vi "Door_Access_System.vi"() -> ()   [LabVIEW 2026]
panel:
  out "String":string
  out "s4":i32
  out "s3":i32
  out "s2":i32
  out "s1":i32
  in  "D":bool
  in  "C":bool
  in  "B":bool
  in  "A":bool
  in  "E":bool
  in  "F":bool
  in  "9":bool
  in  "8":bool
  in  "7":bool
  in  "6":bool
  in  "5":bool
  in  "4":bool
  in  "3":bool
  in  "2":bool
  in  "1":bool
  in  "0":bool
  in  "stop 3":bool
  in  "stop 2":bool
  in  "Digits":i32
  out "7-segment":T1
  in  "stop":bool
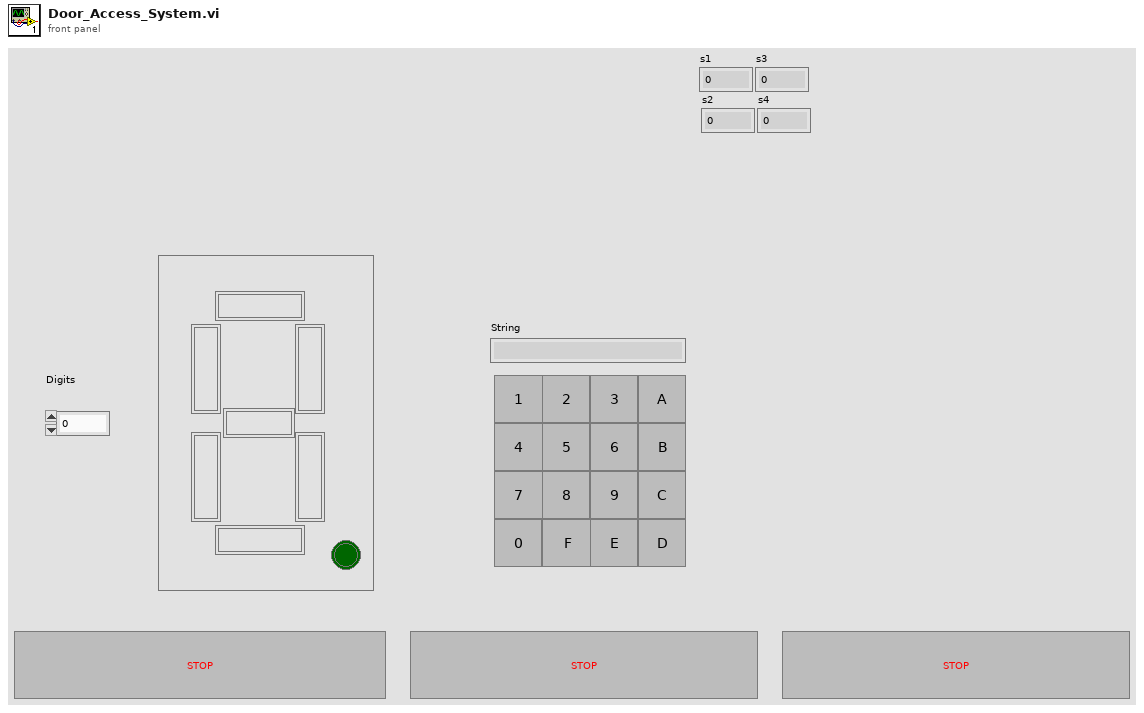
[diagram p1: front panel]
types:
  T1 = cluster{"a":bool, "b":bool, "c":bool, "d":bool, "e":bool, "f":bool, "g":bool, "DP":bool}
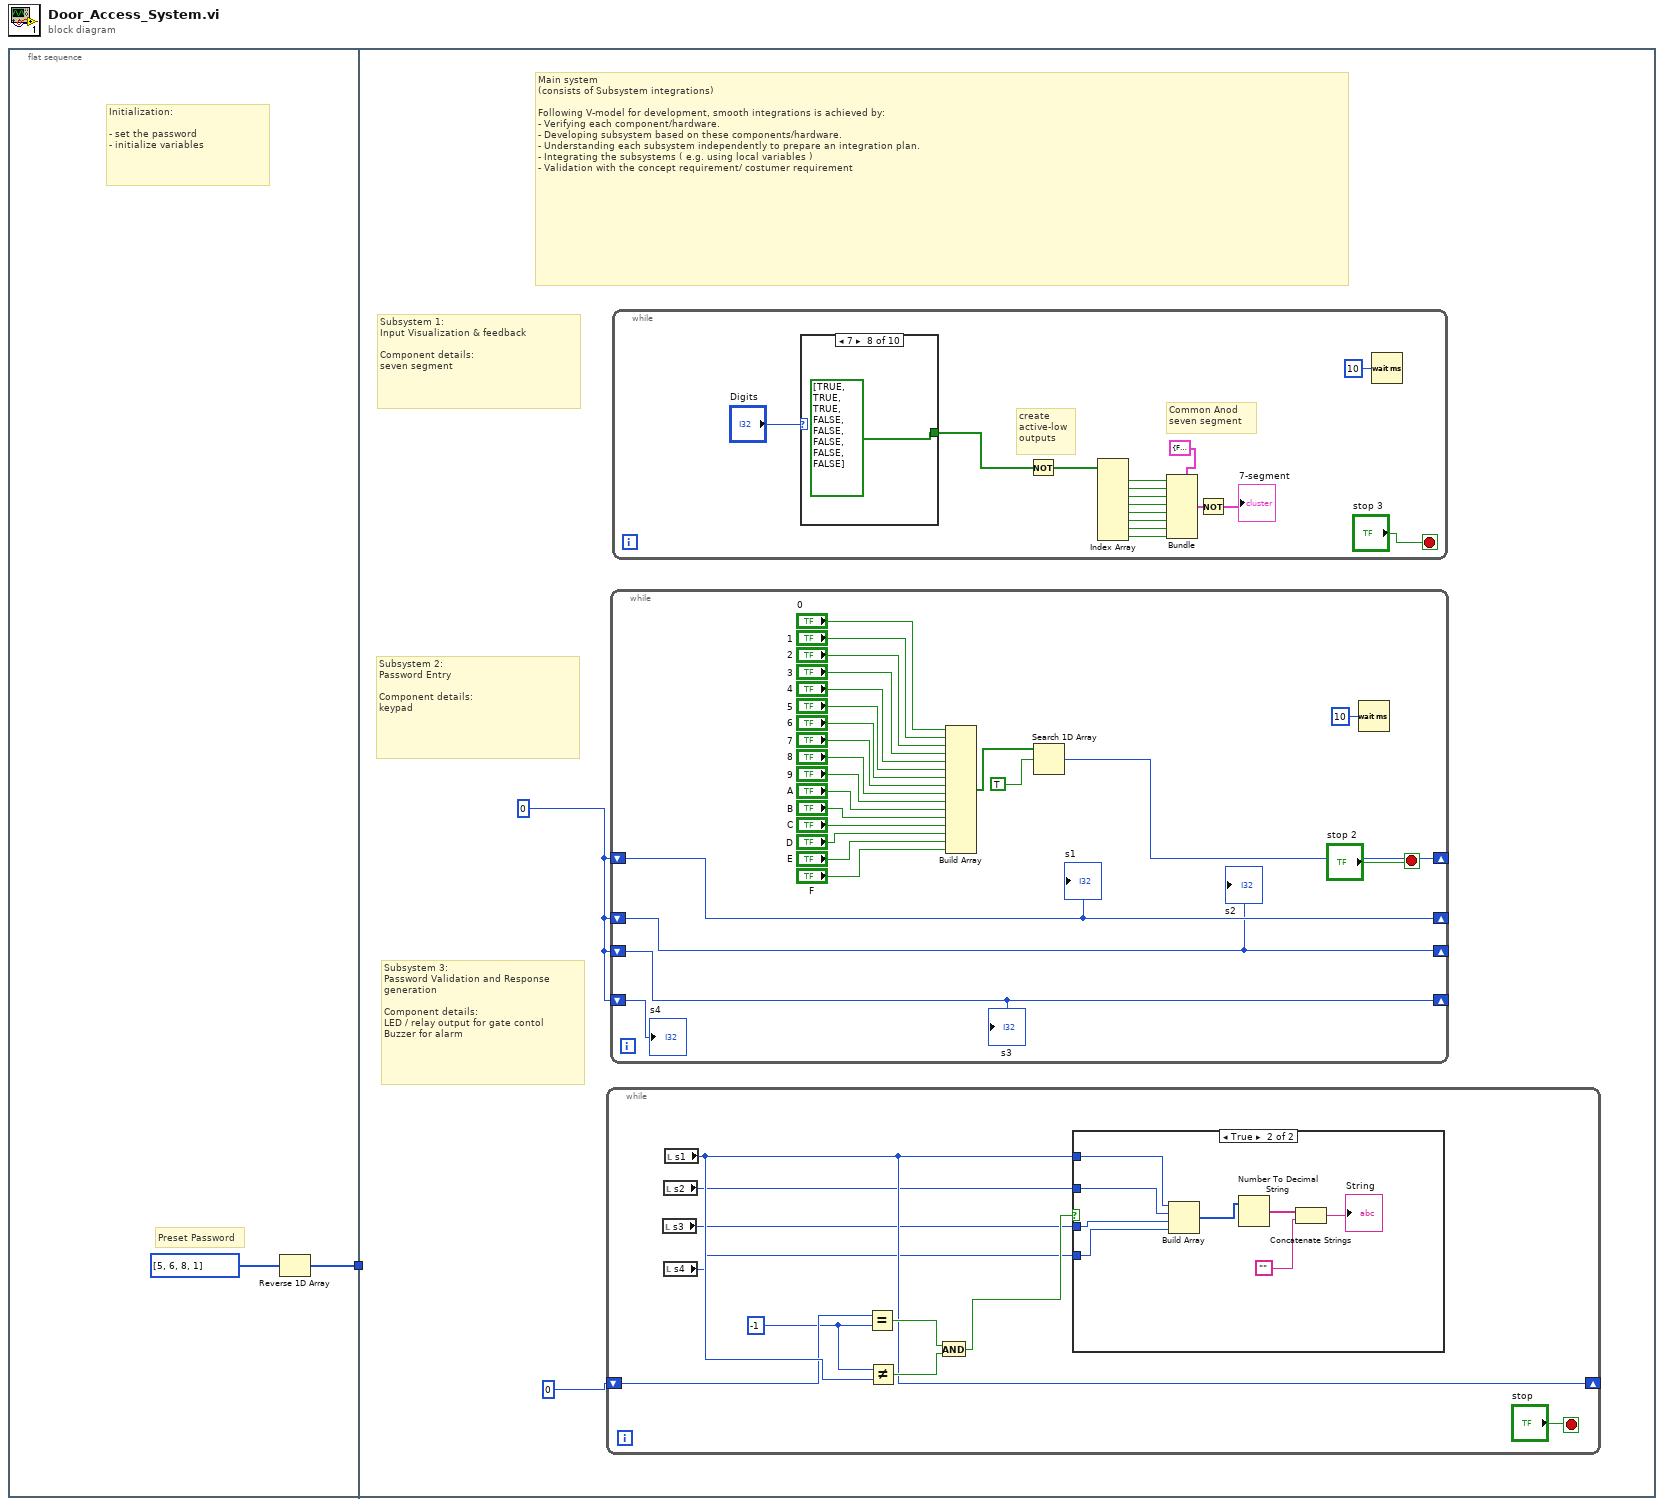
[diagram p0: block diagram]
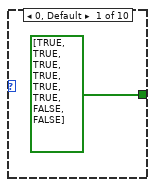
[diagram p2: hidden frame]
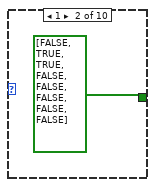
[diagram p3: hidden frame]
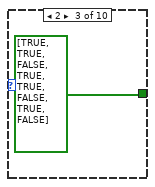
[diagram p4: hidden frame]
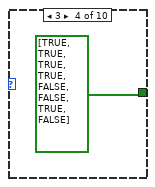
[diagram p5: hidden frame]
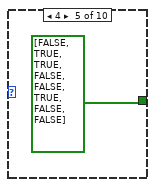
[diagram p6: hidden frame]
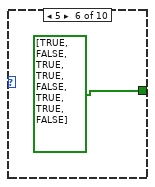
[diagram p7: hidden frame]
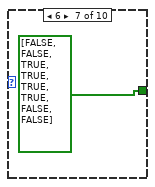
[diagram p8: hidden frame]
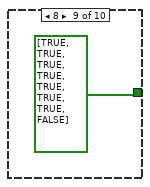
[diagram p9: hidden frame]
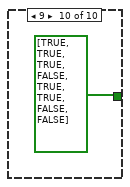
[diagram p10: hidden frame]
diagram:
  n1 = flat-sequence {
    tunnel: [w2] -> w1
    tunnel: w1 -> [_]
    frame #0 {
      # "Preset Password"
      # "Initialization:\n\n- set the password\n- initialize variables"
      n2 = Reverse 1D Array(array=i32[] [5, 6, 8, 1] ("Saved Password")) -> (reversed array=w2:i32[])
    }
    frame #1 {
      w5 = 0
      # "Subsystem 3:\nPassword Validation and Response generation\n\nComponent details:\nLED / relay output for gate contol\nBuzzer for alarm"
      # "Subsystem 1:\nInput Visualization & feedback\n\nComponent details:\nseven segment"
      # "Main system \n(consists of Subsystem integrations)\n\nFollowing V-model for development, smooth integrations is achieved by:\n- Verifying each component/hardware.\n- Developing subsystem based on these components/hardware.\n- Understanding each subsystem independently to prepare an integration plan.\n- Integrating the subsystems ( e.g. using local variables )\n- Validation with the concept requirement/ costumer requirement"
      # "Subsystem 2:\nPassword Entry\n\nComponent details:\nkeypad"
      n3 = while {
        shift-right: [w62] -> _
        shift-left: 0 -> [w61]
        stop <- "stop" stop-if-true
        w57 = -1
        n4 = local read "s3"() -> (w59:i32)
        n5 = local read "s2"() -> (w60:i32)
        n6 = local read "s4"() -> (w58:i32)
        n7 = local read "s1"() -> (w62:i32)
        n8 = Equal?(x=w61, y=w57) -> (x = y?=w64:bool)
        n9 = Not Equal?(x=w57, y=w62) -> (x != y?=w63:bool)
        n10 = And(x=w64, y=w63) -> (x .and. y?=w65:bool)
        n11 = case shown="True" w65 {
          tunnel: w62 -> [_ w74]
          tunnel: w60 -> [_ w73]
          tunnel: w59 -> [_ w72]
          tunnel: w58 -> [_ w71]
          frame False {
          }
          frame True {
            n12 = Build Array(w74, w73, w72, w71) -> (w70:i32[])
            n13 = Number To Decimal String(number=w70) -> (decimal integer string=w69:string[])  [unwired: 1 in]
            n14 = Concatenate Strings(w69, "") -> (→"String":string)
          }
        }
      }
      n15 = while {
        shift-right: [w36] -> _
        shift-left: w5 -> [w35]
        shift-right: [w35] -> _
        shift-left: w5 -> [w34]
        shift-right: [w34] -> _
        shift-left: w5 -> [w33]
        shift-right: [w33] -> _
        shift-left: w5 -> [w32]
        stop <- "stop 2" stop-if-true
        n16 = Build Array("0", "1", "2", "3", "4", "5", "6", "7", "8", "9", "A", "B", "C", "D", "E", "F") -> (w43:bool[])
        n17 = Search 1D Array(1D array=w43, element=TRUE) -> (index of element=w36:i32)  [unwired: 1 in]
        n18 = Wait (ms)(milliseconds to wait=u32 10) -> ()  [unwired: 1 out]
        "s1" <- w35
        "s2" <- w34
        "s3" <- w33
        "s4" <- w32
      }
      n19 = while {
        stop <- "stop 3" stop-if-true
        # "Common Anod \nseven segment"
        # "create\nactive-low\noutputs"
        n20 = case shown="7" "Digits" {
          tunnel: [bool[] [TRUE, TRUE, TRUE, TRUE, TRUE, TRUE, FALSE, FALSE] ("LED segments 2") bool[] [FALSE, TRUE, TRUE, FALSE, FALSE, FALSE, FALSE, FALSE] ("LED segments 2") bool[] [TRUE, TRUE, FALSE, TRUE, TRUE, FALSE, TRUE, FALSE] ("LED segments 2") bool[] [TRUE, TRUE, TRUE, TRUE, FALSE, FALSE, TRUE, FALSE] ("LED segments 2") bool[] [FALSE, TRUE, TRUE, FALSE, FALSE, TRUE, FALSE, FALSE] ("LED segments 2") bool[] [TRUE, FALSE, TRUE, TRUE, FALSE, TRUE, TRUE, FALSE] ("LED segments 2") bool[] [FALSE, FALSE, TRUE, TRUE, TRUE, TRUE, FALSE, FALSE] ("LED segments 2") bool[] [TRUE, TRUE, TRUE, FALSE, FALSE, FALSE, FALSE, FALSE] ("LED segments 2") bool[] [TRUE, TRUE, TRUE, TRUE, TRUE, TRUE, TRUE, FALSE] ("LED segments 2") bool[] [TRUE, TRUE, TRUE, FALSE, TRUE, TRUE, FALSE, FALSE] ("LED segments 2")] -> w20
          frame 0, Default {
          }
          frame 1 {
          }
          frame 2 {
          }
          frame 3 {
          }
          frame 4 {
          }
          frame 5 {
          }
          frame 6 {
          }
          frame 7 {
          }
          frame 8 {
          }
          frame 9 {
          }
        }
        n21 = Not(x=w20) -> (.not. x?=w21:bool[])
        n22 = Index Array "Index Array"(array=w21) -> (element #1=w19:bool, element #2=w18:bool, element #3=w17:bool, element #4=w16:bool, element #5=w15:bool, element #6=w14:bool, element #7=w13:bool, element #8=w12:bool)  [unwired: 8 in]
        n23 = Bundle(cluster=T1 {"a"=FALSE, "b"=FALSE, "c"=FALSE, "d"=FALSE, "e"=FALSE, "f"=FALSE, "g"=FALSE, "DP"=FALSE} ("7-segment"), "a"=w19, "b"=w18, "c"=w17, "d"=w16, "e"=w15, "f"=w14, "g"=w13, "DP"=w12) -> (w10:T1)
        n24 = Not(x=w10) -> (.not. x?=→"7-segment":T1)
        n25 = Wait (ms)(milliseconds to wait=u32 10) -> ()  [unwired: 1 out]
      }
    }
  }
